vi "system_UpdateUserConfig.vi"(8 "error in (no error)":errorcluster, 11 "Config":T1) -> (0 "error out":errorcluster)   [LabVIEW 2013, in "0_SystemCOnfiguration.lvlib"]
uses:
  0_SystemCOnfiguration.lvlib
  system_Config.ctl
  2_Control/ProductType.ctl
  2_Control/PathControl.ctl
panel:
  # "Function Configuration"
  # "Temprary Configuration"
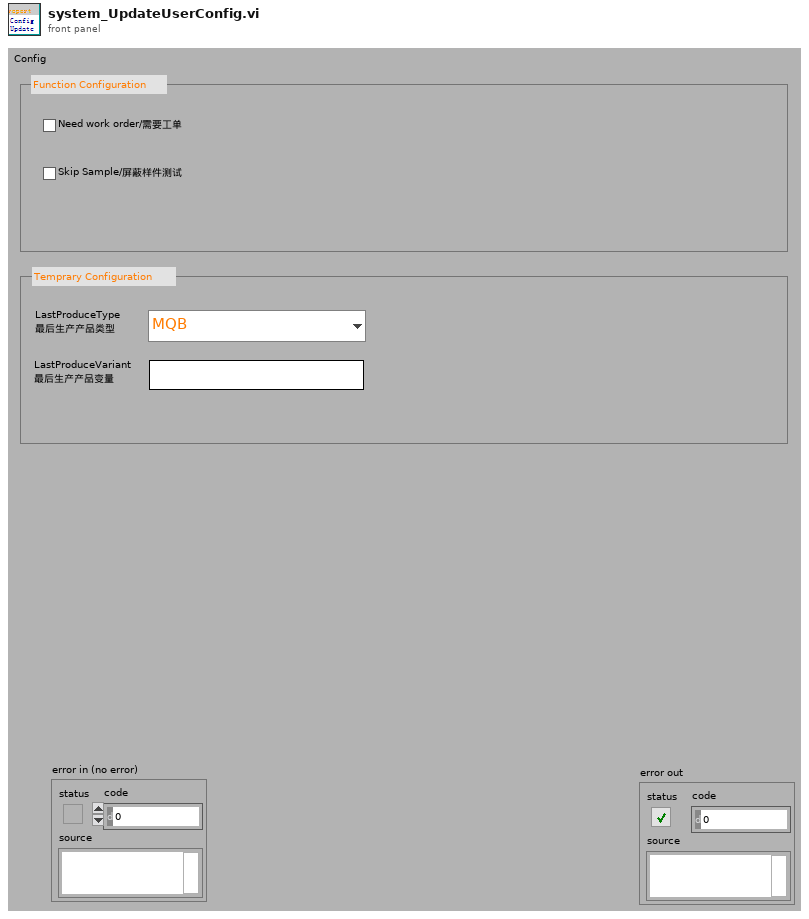
[diagram p1: front panel]
types:
  T1 = typedef "0_SystemCOnfiguration.lvlib/system_Config.ctl" = cluster{"Need work order":bool, "LastTestVariant":string, "Skip Sample":bool, "LastTestType":T2}
  T2 = typedef "ProductType.ctl" = enum16{"MQB", "Geely", "Volvo"}
  T3 = typedef "PathControl.ctl" = enum16{"UI_Banner_Path", "UI_Banner_Path1", "UI_Banner_Path2", "UI_Banner_Path0", "Menu_Manager_Run", "Menu_Debug", "Menu_Operater", "Path_ConfigFolder", "Path_Settings", "Path_Limits", "Path_TestItems", "Path_Company_logo", "Path_UUT", "Path_Customer_logo", "Path_Log_Folder", "Path_Log_Single_Folder", "Path_Config_DB", "Path_TestItem", "Path_TestLimit_Head", "Path_Log_Template", "Path_ExcelLog_Template", "Path_Label", "Path_Manual_Lable", "Path_Manual_TypeConfig", "Path_Message", "Path_ErrorLog_Folder"}
  T4 = typedef "system_Config.ctl" = cluster{"Need work order":bool, "LastTestVariant":string, "Skip Sample":bool, "LastTestType":T2}
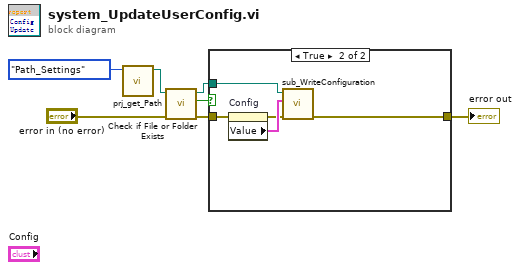
[diagram p0: block diagram]
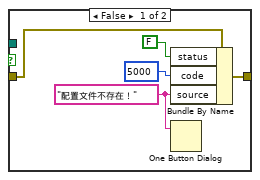
[diagram p2: hidden frame]
diagram:
  n1 = call "prj_get_Path.vi"("Path_Item"=PathControl."Path_Settings") -> ("Detail path"=w2:path)  [unwired: 10 in]
  n2 = call <vilib>:"Check if File or Folder Exists.vi"("error in (no error)"="error in (no error)", "path"=w2) -> ("error out"=w5:errorcluster, "file or folder exists?"=w7:bool, "dup path"=w6:path)  [unwired: 7 in]
  n3 = case shown="True" w7 {
    tunnel: w6 -> [_ w16]
    tunnel: w5 -> [w12 w14]
    tunnel: [w11 w17] -> w4
    frame False {
      w9 = "配置文件不存在！" ("消息")
      n4 = Bundle By Name(cluster=w12, "status"=FALSE, "code"=5000, "source"=w9) -> (w11:errorcluster)
      n5 = One Button Dialog(message=w9) -> ()  [unwired: 1 in, 1 out]
    }
    frame True {
      n6 = property on="Config" class="Clust (strict)"(error in=w14) -> (error out=w13:errorcluster, "Value"=w15:T4)  [unwired: 1 in, 1 out]
      n7 = call "sub_WriteConfiguration.vi"("error in (no error)"=w13, "INI Fomatted Cluster"=w15, "configuration file path"=w16) -> ("error out"=w17:errorcluster)  [unwired: 8 in]
    }
  }
  "error out" <- w4
